vi "Step Core.vi"(8 "error in (no error)":errorcluster, 11 "Skyworks - 2G PVT in":refnum<class "Skyworks - PVT.lvclass">) -> (0 "error out":errorcluster, 3 "Skyworks - 2G PVT out":refnum<class "Skyworks - PVT.lvclass">)   [LabVIEW 2018, in "Skyworks PVT.lvlib" / "Skyworks - PVT.lvclass"]
uses:
  Skyworks - PVT.lvclass
  Plugins/Measurement Interface.lvlibp/Measurement Interface.lvclass
  C:/Sequence Automation/Plugins/Measurement Interface.lvlibp/Measurement Interface.lvclass
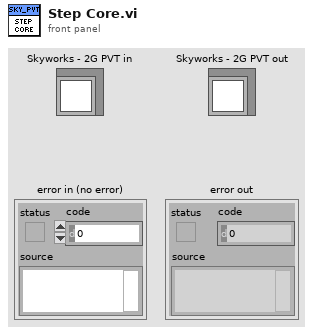
[diagram p1: front panel]
types:
  T1 = typedef "TestStand API Tools (TSAT).lvlibp/TSAT Evaluation Actions.lvlib/TSAT Evaluation.ctl" = cluster{"Test Name":string, "Pin":string, "Units":string, "SI Scaling":T2, "Test Number":i32, "Published Data Id":string, "Low Limit":dbl, "High Limit":dbl, "Export Data Location":string, "Software Bin":i64, "Evaluation Type":T3, "Test Data Source":string}
  T2 = typedef "TestStand API Tools (TSAT).lvlibp/TSAT Evaluation Actions.lvlib/TSAT Eval SI Unit Scaling.ctl" = i16
  T3 = typedef "TestStand API Tools (TSAT).lvlibp/TSAT Evaluation Actions.lvlib/TSAT Evaluation Type.ctl" = enum16{"Numeric Limit", "Pass/Fail", "None"}
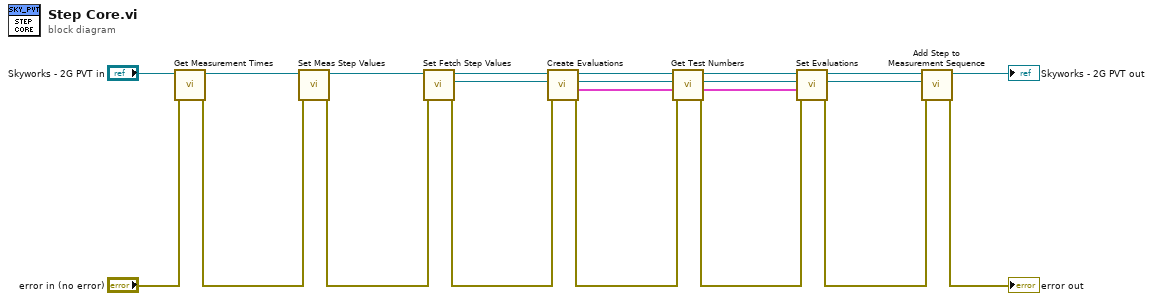
[diagram p0: block diagram]
diagram:
  n1 = call "Get Measurement Times.vi"("error in (no error)"="error in (no error)", "Skyworks - 2G PVT in"="Skyworks - 2G PVT in") -> ("error out"=w3:errorcluster, "Skyworks - 2G PVT out"=w4:refnum<class "Skyworks - PVT.lvclass">)  [unwired: 8 in]
  n2 = call "Set Meas Step Values.vi"("error in (no error)"=w3, "Skyworks - PVT in"=w4) -> ("error out"=w2:errorcluster, "Skyworks - PVT out"=w1:refnum<class "Skyworks - PVT.lvclass">)  [unwired: 8 in]
  n3 = call "Set Fetch Step Values.vi"("error in (no error)"=w2, "Skyworks - 2G PVT in"=w1) -> ("error out"=w17:errorcluster, "Fetch Step Out"=w10:refnum<k7>, "Skyworks - 2G PVT out"=w18:refnum<class "Skyworks - PVT.lvclass">)  [unwired: 7 in]
  n4 = call-dynamic "Create Evaluations.vi"("error in (no error)"=w17, "Skyworks - 2G PVT in"=w18) -> ("error out"=w15:errorcluster, "Evaluations Out"=w12:T1[], "Skyworks - 2G PVT out"=w16:refnum<class "Skyworks - PVT.lvclass">)  [unwired: 7 in]
  n5 = call "Get Test Numbers.vi"("error in (no error)"=w15, "Evaluations In"=w12, "Skyworks - 2G PVT in"=w16) -> ("error out"=w13:errorcluster, "Evaluations Out"=w11:T1[], "Skyworks - 2G PVT out"=w14:refnum<class "Skyworks - PVT.lvclass">)  [unwired: 6 in]
  n6 = call "Set Evaluations.vi"("error in (no error)"=w13, "Evaluation Data"=w11, "Step In"=w10, "Skyworks - 2G PVT in"=w14) -> ("error out"=w7:errorcluster, "Step Out"=w8:refnum<k7>, "Skyworks - 2G PVT out"=w9:refnum<class "Skyworks - PVT.lvclass">)  [unwired: 5 in]
  n7 = call "Add Step to Measurement Sequence.vi"("error in (no error)"=w7, "Step to Add"=w8, "Measurement Interface in"=w9) -> ("error out"=→"error out":errorcluster, "Measurement Interface out"=→"Skyworks - 2G PVT out":refnum<class "Skyworks - PVT.lvclass">)  [unwired: 7 in]
